vi "TriangleScan(Two axis).vi"() -> ()   [LabVIEW 2012]
uses:
  Madlib.dll
panel:
  out "Y Position (um)":dbl(graph)
  in  "Y DELAY (ms)":u32=30
  in  "Y Samples":u16=100 min=1 step=1
  in  "Y End  (um)":dbl=100.0 min=0.0 max=100.0 step=0.2 format="%.3f"
  in  "Y Start  (um)":dbl min=0.0 max=100.0 step=0.5 format="%.3f"
  in  "X DELAY (ms)":u32=10
  out "X Position (um)":dbl(graph)
  in  "X Samples":u16=100 min=1 step=1
  in  "X Start  (um)":dbl min=0.0 max=100.0 step=0.5 format="%.3f"
  in  "X End  (um)":dbl=100.0 min=0.0 max=100.0 step=0.2 format="%.3f"
  # "This VI implements a triangle scan in X and Y.  For each step in the linear ramp in Y the X axis is stepped through its \nentire linear ramp.  When the X axis reachs the end of its ramp Y is stepped and the linear ramp for X is inverted.\nIt is important to note that this type of scan can lead to phase shift issues.  Basically if the nanopositioner does\nnot settle after each step it will *lag* behind the latest control position and on the return the *lag* will be in the\n other direction. So you may read 0-99 in one direction and 100 - 1 in the other direction."
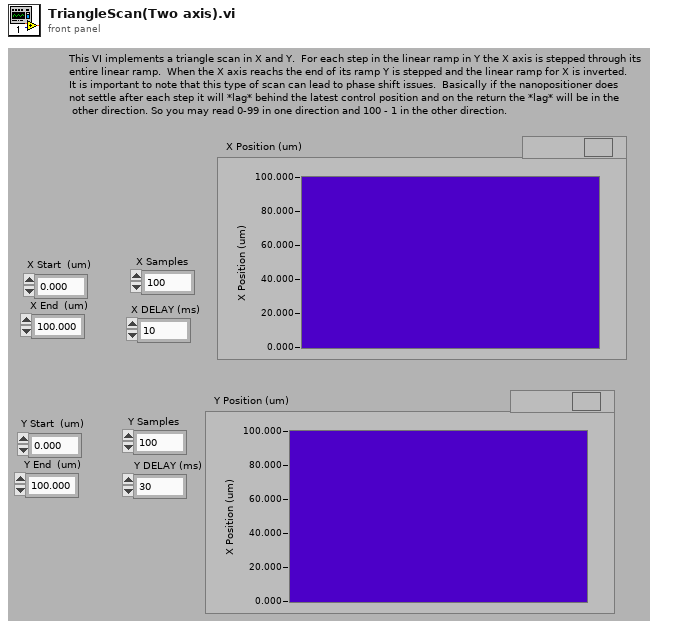
[diagram p1: front panel]
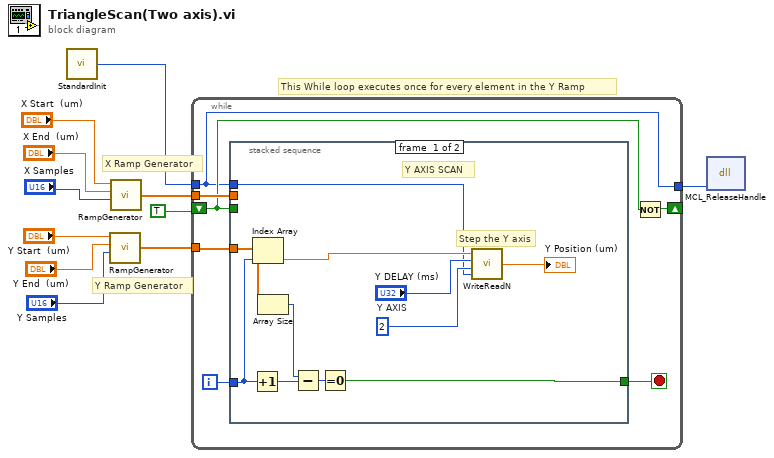
[diagram p0: block diagram]
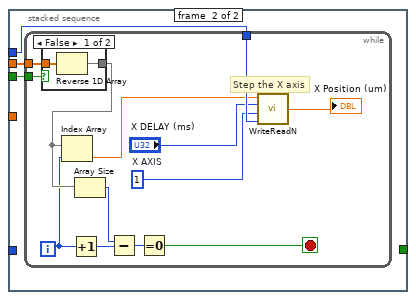
[diagram p2: hidden frame]
diagram:
  # "This While loop executes once for every element in the Y Ramp"
  # "X Ramp Generator"
  # "Y Ramp Generator"
  n1 = call "StandardInit.vi"() -> ("Outgoing Handle"=w2:i32)  [unwired: 1 in]
  n2 = call "RampGenerator.vi"("Number of Positions"="Y Samples", "End  (um)"="Y End  (um)", "Start  (um)"="Y Start  (um)") -> ("Array"=w3:dbl[])  [unwired: 1 in]
  n3 = call "RampGenerator.vi"("Number of Positions"="X Samples", "End  (um)"="X End  (um)", "Start  (um)"="X Start  (um)") -> ("Array"=w11:dbl[])  [unwired: 1 in]
  n4 = while {
    tunnel: w11 -> [w16]
    tunnel: w3 -> [w13]
    shift-right: [w14] -> _
    shift-left: TRUE -> [w15]
    tunnel: w2 -> [w12]
    tunnel: [w12] -> w1
    i -> [w17]
    stop <- w18 stop-if-true
    # "X Ramp Generator"
    n5 = stacked-sequence {
      tunnel: w13 -> [w28 _]
      tunnel: [w26 _] -> w18
      tunnel: w17 -> [w25 _]
      tunnel: w16 -> [_ w32]
      tunnel: w15 -> [_ w31]
      tunnel: w12 -> [w19 w30]
      frame #0 {
        w20 = 2  # Y AXIS
        # "Step the Y axis"
        # "Y AXIS SCAN"
        n6 = Increment(x=w25) -> (x+1=w24:i32)
        n7 = Index Array(array=w28, index=w25) -> (element=w22:dbl)
        n8 = Array Size(array=w28) -> (size(s)=w27:i32)
        n9 = Subtract(x=w27, y=w24) -> (x-y=w29:i32)
        n10 = Equal To 0?(x=w29) -> (x = 0?=w26:bool)
        n11 = call "WriteReadN.vi"("Handle"=w19, "Axis"=w20, "Delay (ms)"="Y DELAY (ms)", "Move to (um)"=w22) -> ("Current Position (um)"=→"Y Position (um)":dbl)
      }
      frame #1 {
        n12 = while {
          tunnel: w32 -> [w44]
          tunnel: w31 -> [w42]
          tunnel: w30 -> [w36]
          i -> [w37]
          stop <- w40 stop-if-true
          w33 = 1  # X AXIS
          # "Step the X axis"
          n13 = case shown="False" w42 {
            tunnel: w44 -> [w46 w48]
            tunnel: [w47 w48] -> w43
            frame False {
              n14 = Reverse 1D Array(array=w46) -> (reversed array=w47:dbl[])
            }
            frame True {
            }
          }
          n15 = Index Array(array=w43, index=w37) -> (element=w35:dbl)
          n16 = Increment(x=w37) -> (x+1=w38:i32)
          n17 = Array Size(array=w43) -> (size(s)=w41:i32)
          n18 = Subtract(x=w41, y=w38) -> (x-y=w45:i32)
          n19 = Equal To 0?(x=w45) -> (x = 0?=w40:bool)
          n20 = call "WriteReadN.vi"("Handle"=w36, "Axis"=w33, "Delay (ms)"="X DELAY (ms)", "Move to (um)"=w35) -> ("Current Position (um)"=→"X Position (um)":dbl)
        }
      }
    }
    n21 = Not(x=w15) -> (.not. x?=w14:bool)
  }
  n22 = dll-call lib="C:/Users/Labview/Desktop/SRR/Madlib_x64/Labview Examples/MADLib.dll" fn="MCL_ReleaseHandle"("handle"=w1) -> ()  [unwired: 5 in, 2 out]
